vi "Configure MCCW Crest Factor Mode.vi"(8 "error in (no error)":errorcluster, 9 "Crest factor target":dbl, 10 "Crest factor mode":enum16{"Off", "Chirp", "Slow"}(ring), 11 "Vector Signal Generator in":refnum<class "Vector Signal Generator.lvclass">) -> (0 "error out":errorcluster, 3 "Vector Signal Generator out":refnum<class "Vector Signal Generator.lvclass">)   [LabVIEW 2020, in "Vector Signal Generator.lvclass"]
doc: "Configure the crest factor optimazation mode"
uses:
  Vector Signal Generator.lvclass
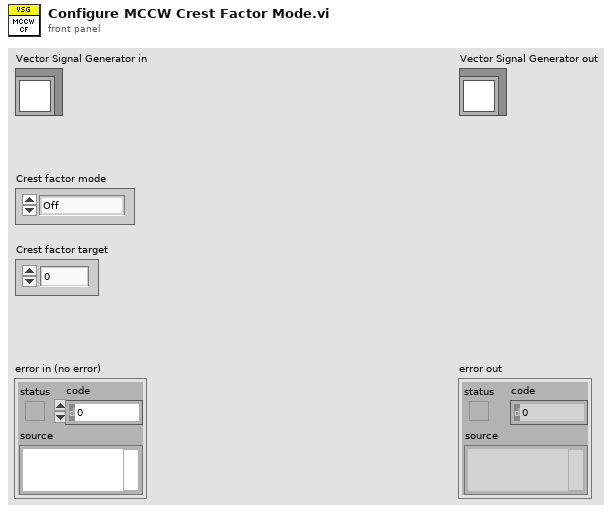
[diagram p1: front panel]
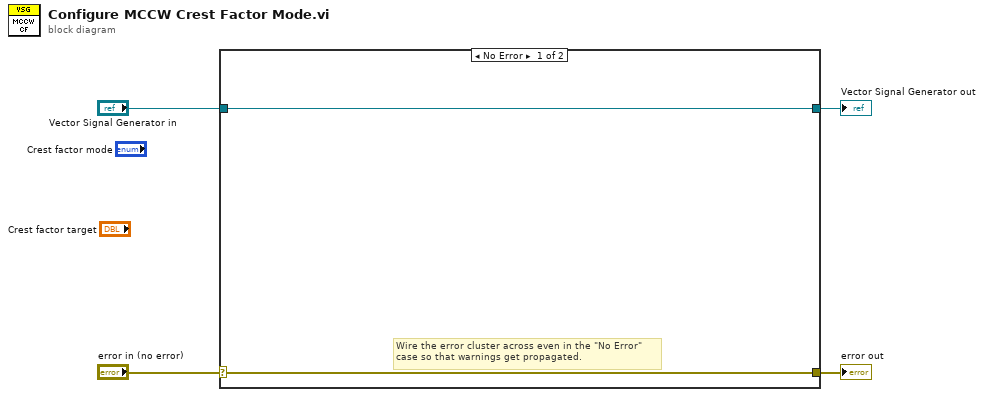
[diagram p0: block diagram]
diagram:
  n1 = case shown="No Error" "error in (no error)" {
    selector: "error in (no error)" -> [w5 w8]
    tunnel: [w5 w8] -> w3
    tunnel: [w6 w7] -> w1
    tunnel: "Vector Signal Generator in" -> [w6 w7]
    frame No Error {
      # "Wire the error cluster across even in the \"No Error\"\ncase so that warnings get propagated."
    }
    frame Error {
    }
  }
  "error out" <- w3
  "Vector Signal Generator out" <- w1
